vi "WriteEvtConfig.vi"(8 "error in (no error)":errorcluster, 10 "Event Configuration":T1={"UTC Time 0"=timestamp(0 s since 1904-01-01), "Nominal Frequency"=60, "Reporting Rate"=60, "Fsamp"=960, "PosSeq"=FALSE} {"Reporting Rate" items=["10 FPS"=10, "12 FPS"=12, "15 FPS"=15, "20 FPS"=20, "25 FPS"=25, "30 FPS"=30, "50 FPS"=50, "60 FPS"=60]; "Nominal Frequency" items=["50 Hz"=50, "60 Hz"=60]}, 11 "RingdownPlugin in":refnum<class "EraPlugin.lvclass">) -> (0 "error out":errorcluster, 3 "RingdownPlugin out":refnum<class "EraPlugin.lvclass">)   [LabVIEW 2017, in "AppPlugins.lvlib" / "ERAPlugin.lvclass"]
uses:
  EraPlugin.lvclass
  Framework/FrontPanel/TypeDefs/clEventConfig.ctl
  EraPlugin.lvclass/EraPlugin.ctl
  Accessors/Read RingdownConfig.vi
  Framework/Framework.lvlib
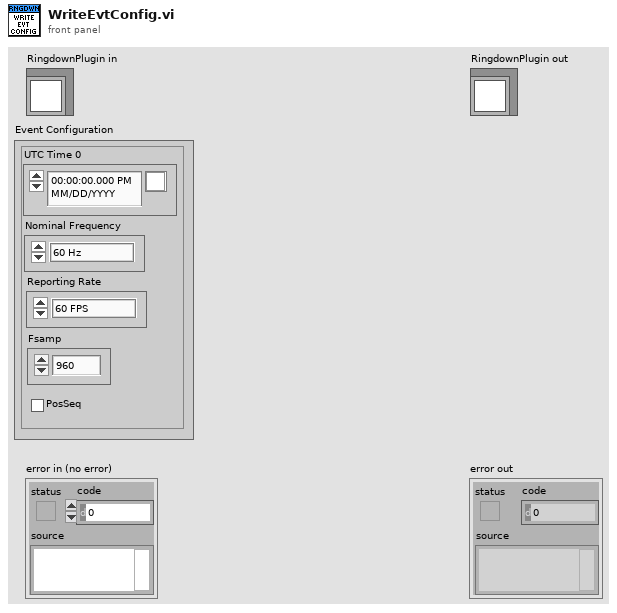
[diagram p1: front panel]
types:
  T1 = typedef "Framework.lvlib/clEventConfig.ctl" = cluster{"UTC Time 0":timestamp, "Nominal Frequency":u16, "Reporting Rate":u16, "Fsamp":u32, "PosSeq":bool}
  T2 = typedef "AppPlugins.lvlib/ERAPlugin.lvclass/RingdownConfig.ctl" = cluster{"Config":cluster{"p_SysOdr":i32, "dThres":dbl, "Preproc":cluster{"order":i32, "f_lo":dbl, "f_hi":dbl, "R_down":i32}}, "V index":i32, "I index":i32, "PosSeq":bool}
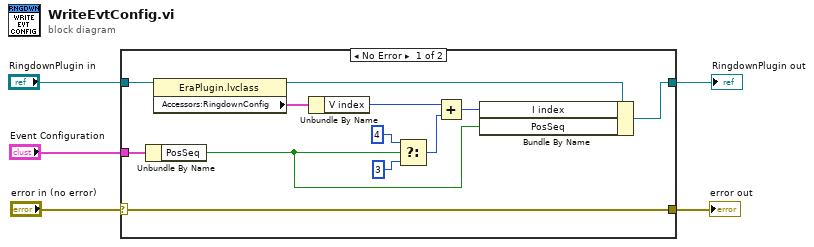
[diagram p0: block diagram]
diagram:
  n1 = case shown="No Error" "error in (no error)" {
    selector: "error in (no error)" -> [w7 w18]
    tunnel: "RingdownPlugin in" -> [w16 w19]
    tunnel: [w8 w19] -> w3
    tunnel: [w7 w18] -> w2
    tunnel: "Event Configuration" -> [w17 _]
    frame No Error {
      n2 = Unbundle By Name(w17) -> ("PosSeq"=w6:bool)
      n3 = property class="EraPlugin.lvclass"(reference=w16) -> (reference out=w10:refnum<class "EraPlugin.lvclass">, "Accessors:RingdownConfig"=w15:T2)  [unwired: 1 in, 1 out]
      n4 = Unbundle By Name(w15) -> ("V index"=w11:i32)
      n5 = Select(t=4, s=w6, f=3) -> (s? t:f=w12:i32)
      n6 = Add(x=w11, y=w12) -> (x+y=w9:i32)
      n7 = Bundle By Name(cluster=w10, "I index"=w9, "PosSeq"=w6) -> (w8:refnum<class "EraPlugin.lvclass">)
    }
    frame Error {
    }
  }
  "error out" <- w2
  "RingdownPlugin out" <- w3
